vi "Send RDS Child Receive Message.vi"(7 "Priority":T1=enum."Normal" caption="Message Priority (Normal)", 8 "error in (no error)":errorcluster, 10 "RDS Message":refnum<class "RDS Message.lvclass">, 11 "Message Enqueuer in":refnum<class "Message Enqueuer.lvclass">) -> (0 "error out":errorcluster, 3 "Message Enqueuer out":refnum<class "Message Enqueuer.lvclass">)   [LabVIEW 2015, in "RDS Abstracts.lvlib" / "RDS Parent Actor.lvlib" / "RDS Child Receive Message Msg.lvclass"]
doc: "Sends the <b>RDS Child Receive Message Msg.lvclass</b> message.\n\nThis message will call <b>RDS Child Receive Message.vi</b> on the <b>RDS Parent Actor.lvlib:RDS Parent Actor.lvclass</b> actor.\n\n<b>RDS Child Receive Message.vi Description</b>"
uses:
  RDS Child Receive Message Msg.lvclass
  <vilib>/ActorFramework/Message Enqueuer/Message Enqueuer.lvclass
  <vilib>/ActorFramework/Message Enqueuer/Message Priority.ctl
  Libraries/RDS Framework/RDS Message Class/RDS Message.lvclass
  RDS Child Receive Message Msg.lvclass/RDS Child Receive Message Msg.ctl
  <vilib>/ActorFramework/Message Enqueuer/Message Enqueuer.lvclass/Message Enqueuer.ctl
  <vilib>/ActorFramework/Message Priority Queue/Priority Enqueue.vi
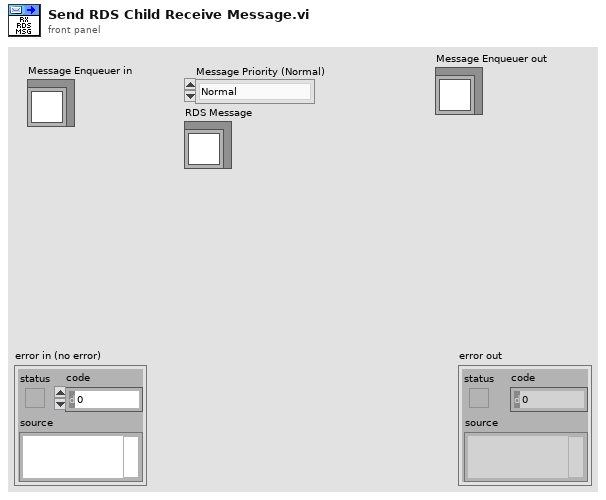
[diagram p1: front panel]
types:
  T1 = typedef "Actor Framework.lvlib/Message Enqueuer.lvclass/Message Priority.ctl" = enum16{"Low", "Normal", "High"}
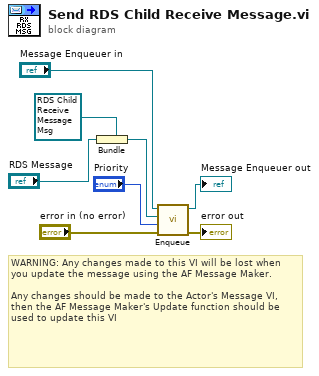
[diagram p0: block diagram]
diagram:
  # "WARNING: Any changes made to this VI will be lost when you update the message using the AF Message Maker.\n\nAny changes should be made to the Actor's Message VI, then the AF Message Maker's Update function should be used to update this VI"
  n1 = Bundle(cluster=refnum<class "RDS Child Receive Message Msg.lvclass"> refnum ("RDS Child Receive Message Msg.lvclass"), "RDS Message") -> (w4:refnum<class "RDS Child Receive Message Msg.lvclass">)
  n2 = call <vilib>:"Enqueue.vi"("error in (no error)"="error in (no error)", "Message Priority (Normal)"="Priority", "Message"=w4, "Message Enqueuer in"="Message Enqueuer in") -> ("error out"=→"error out":errorcluster, "Message Enqueuer out"=→"Message Enqueuer out":refnum<class "Message Enqueuer.lvclass">)  [unwired: 6 in]
